vi "Find Device By Serial.vi"(8 "error in":errorcluster, 11 "IMG_SRC in":refnum<class "IMG_SRC.lvclass">) -> (0 "error out":errorcluster, 3 "IMG_SRC out":refnum<class "IMG_SRC.lvclass">)   [LabVIEW 2018, in "IMG_SRC.lvlib" / "IMG_SRC.lvclass"]
uses:
  IMG_SRC.lvclass
  IMG_SRC.lvclass/IMG_SRC.ctl
  builds/Camera.lvlibp/Camera.lvclass
  C:/Users/Ron.Dexter.LUMINARTECH/Desktop/builds/Camera.lvlibp/Camera.lvclass
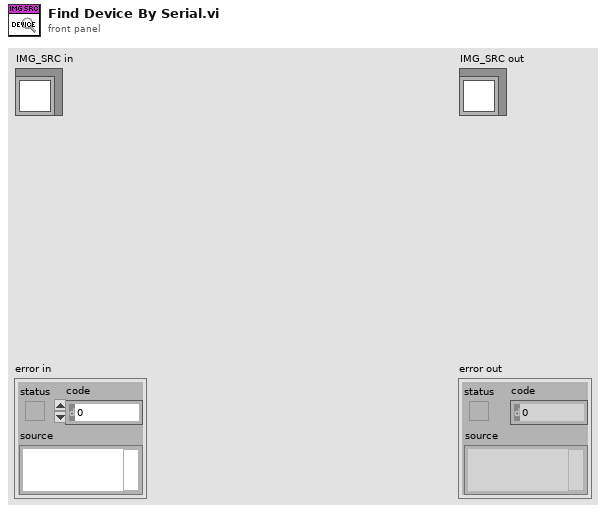
[diagram p1: front panel]
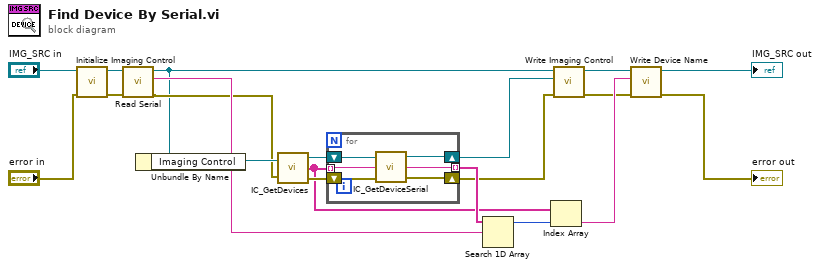
[diagram p0: block diagram]
diagram:
  n1 = call "Initialize Imaging Control.vi"("error in"="error in", "IMG_SRC in"="IMG_SRC in") -> ("error out"=w13:errorcluster, "IMG_SRC out"=w12:refnum<class "IMG_SRC.lvclass">)  [unwired: 8 in]
  n2 = call "Read Serial.vi"("error in (no error)"=w13, "Camera in"=w12) -> ("error out"=w9:errorcluster, "Serial"=w11:string, "Camera out"=w7:refnum<class "IMG_SRC.lvclass">)  [unwired: 7 in]
  n3 = Unbundle By Name(w7) -> ("Imaging Control"=w10:refnum<k7>)
  n4 = call <userlib>:"IC_GetDevices.vi"("ICImagingControl In"=w10, "Error In (no error)"=w9) -> ("ICImagingControl Out"=w20:refnum<k7>, "Devices"=w14:string[], "Error Out"=w19:errorcluster)
  n5 = for {
    tunnel: w14 -> [w24] mode=indexing
    shift-right: [w23] -> w6
    shift-left: w20 -> [w25]
    shift-right: [w22] -> w1
    shift-left: w19 -> [w26]
    tunnel: [w21] -> w15 mode=indexing
    n6 = call <userlib>:"IC_GetDeviceSerial.vi"("Error In (no error)"=w26, "Device"=w24, "ICImagingControl In"=w25) -> ("Error Out"=w22:errorcluster, "Serial"=w21:string, "ICImagingControl Out"=w23:refnum<k7>)
  }
  n7 = Search 1D Array(1D array=w15, element=w11) -> (index of element=w16:i32)  [unwired: 1 in]
  n8 = Index Array(array=w14, index=w16) -> (element=w5:string)
  n9 = call "Write Imaging Control.vi"("error in (no error)"=w1, "Imaging Control"=w6, "IMG_SRC in"=w7) -> ("error out"=w2:errorcluster, "IMG_SRC out"=w8:refnum<class "IMG_SRC.lvclass">)  [unwired: 7 in]
  n10 = call "Write Device Name.vi"("error in (no error)"=w2, "Device Name"=w5, "IMG_SRC in"=w8) -> ("error out"=→"error out":errorcluster, "IMG_SRC out"=→"IMG_SRC out":refnum<class "IMG_SRC.lvclass">)  [unwired: 7 in]
